vi "Plugin-002-CalibrationTest.vi"(0 "Configuration Page":refnum<class "Material-ConfigPage.lvclass">, 11 "error in":errorcluster) -> (15 "error out":errorcluster)   [LabVIEW 2013, in "Calibration-RunTest.lvclass"]
doc: "DisplayName=\"Deploy Configuration Template\"\nDescription=\"This VI serves as a template page for the Deploy Configuration UI.\""
uses:
  Plugins/Run Calibration Test/Calibration-RunTest.lvclass
  Material-ConfigPage.lvclass
  Reuse Library/featherweight/Core/Sequencer/FTW-Sequencer.lvclass/FTW-Sequencer.ctl
  Plugins/Run Calibration Test/Calibration-RunTest.lvclass/Calibration-RunTest.ctl
  <vilib>/Utility/miscctls.llb/LVPointTypeDef.ctl
  Reuse Library/featherweight/Core/Regex/FTW-Regex.vi
  Reuse Library/featherweight/Core/Error/FTW-ERR-StatusException.vi
  Reuse Library/featherweight/Core/Error/FTW-ERR-ThrowError.vi
  Reuse Library/featherweight/Core/Sequencer/FTW-Sequencer.lvclass
  Reuse Library/featherweight/Core/Messaging/Message.Actor/FTW-Message-Actor.lvclass
  Plugins/Motion Control/Motion-ControlAll.lvclass
  <instrlib>/Keyence LK-G5000/Keyence LK-G5000.lvlib
  <instrlib>/Keyence LK-G5000/Public/Constant/Comm Interface.ctl
  <vilib>/addons/_LabVIEW Style Book/Utilities/Style Book Utilities.lvlib
panel:
  out "Calibration Complete":bool
  in  "Collect Cal Data":bool
  out "Line 3 Calibration Data":dbl[](graph)
  out "Line 2 Calibration Data":dbl[](graph)
  out "Line 1 Calibration Data":dbl[](graph)
  # "Inputs"
  # "Outputs"
  # "Second Plugin"
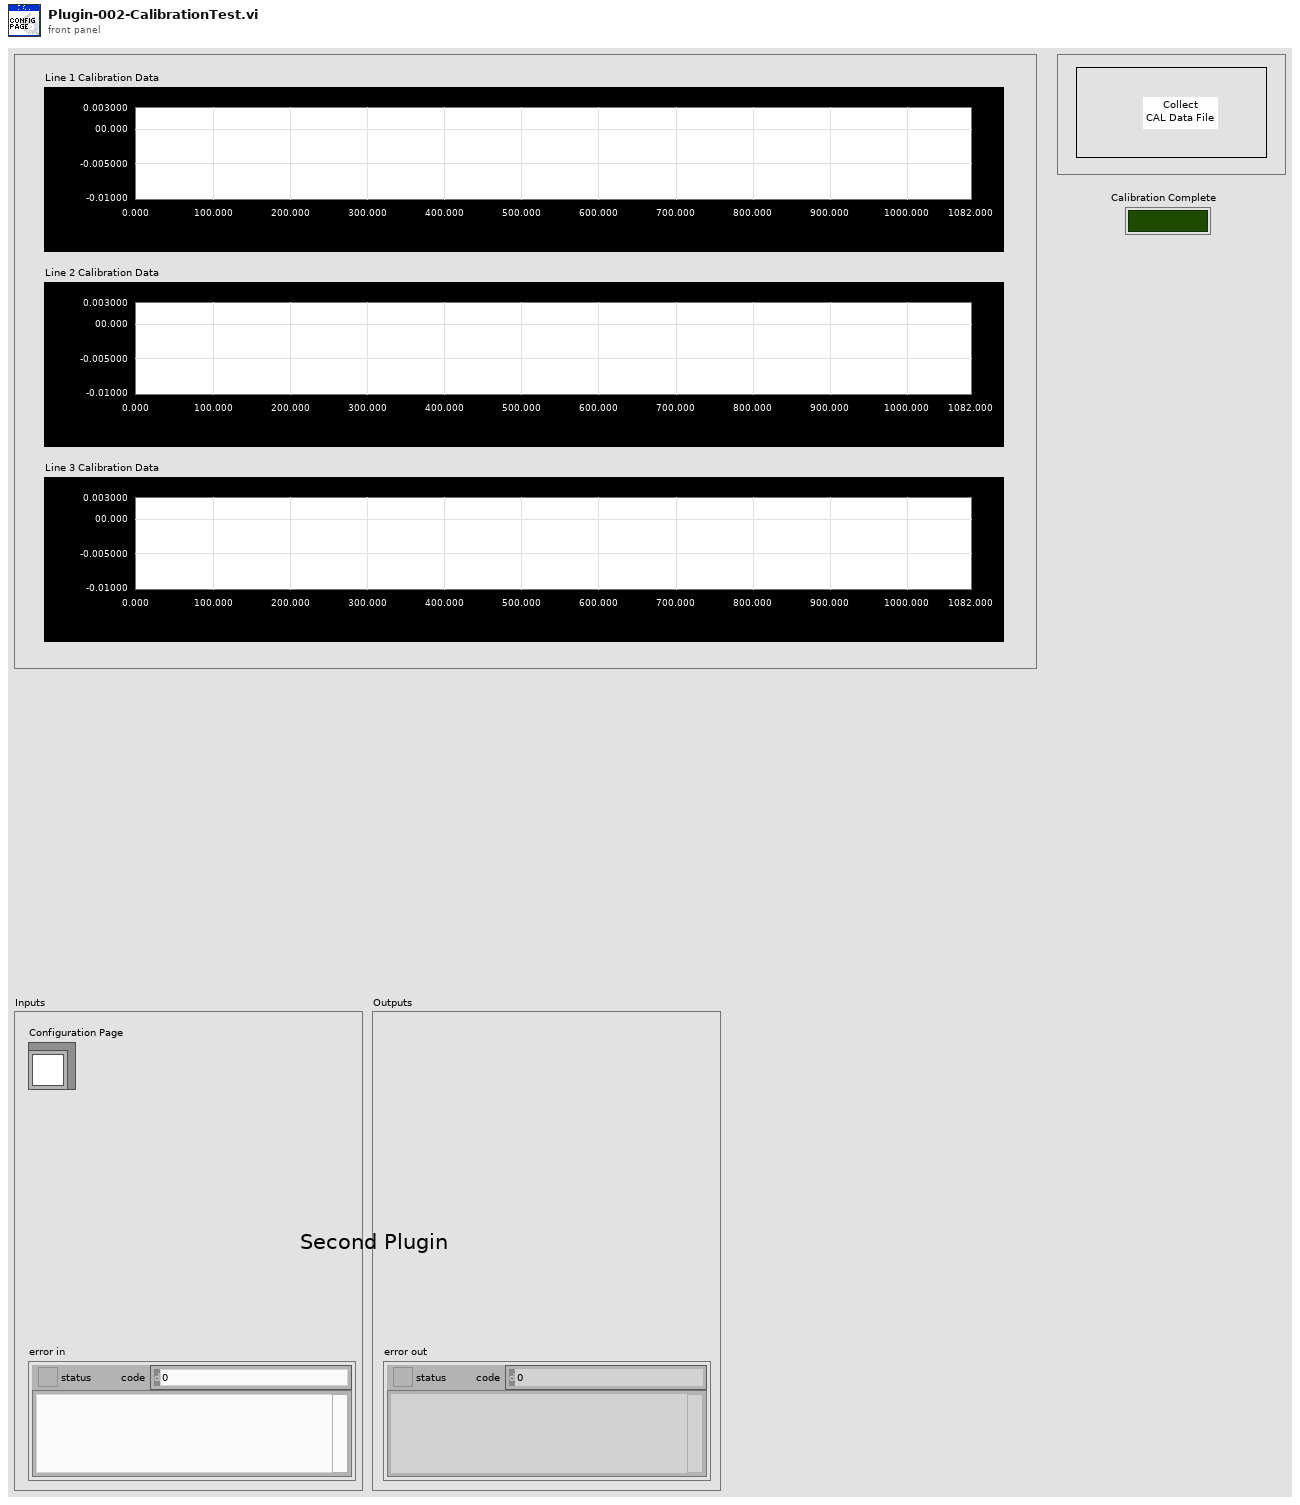
[diagram p1: front panel]
types:
  T1 = typedef "Keyence LK-G5000.lvlib/Comm Interface.ctl" = enum8{"USB", "ETHERNET"}
  T2 = typedef "LVPointTypeDef.ctl" = cluster{"Horizontal":i16, "Vertical":i16}
  T3 = cluster{"PageCommands":refnum<event-registration>}
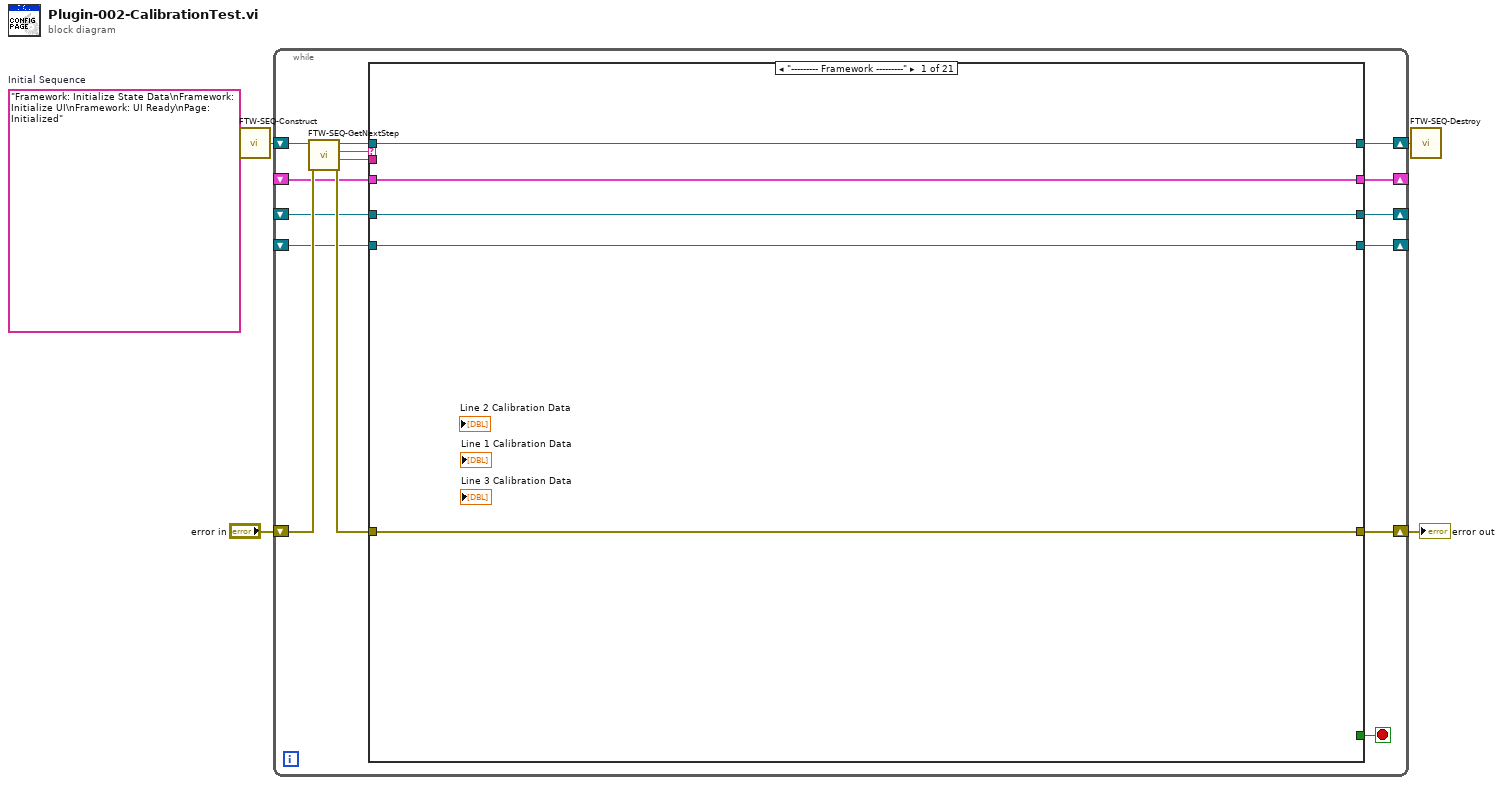
[diagram p0: block diagram]
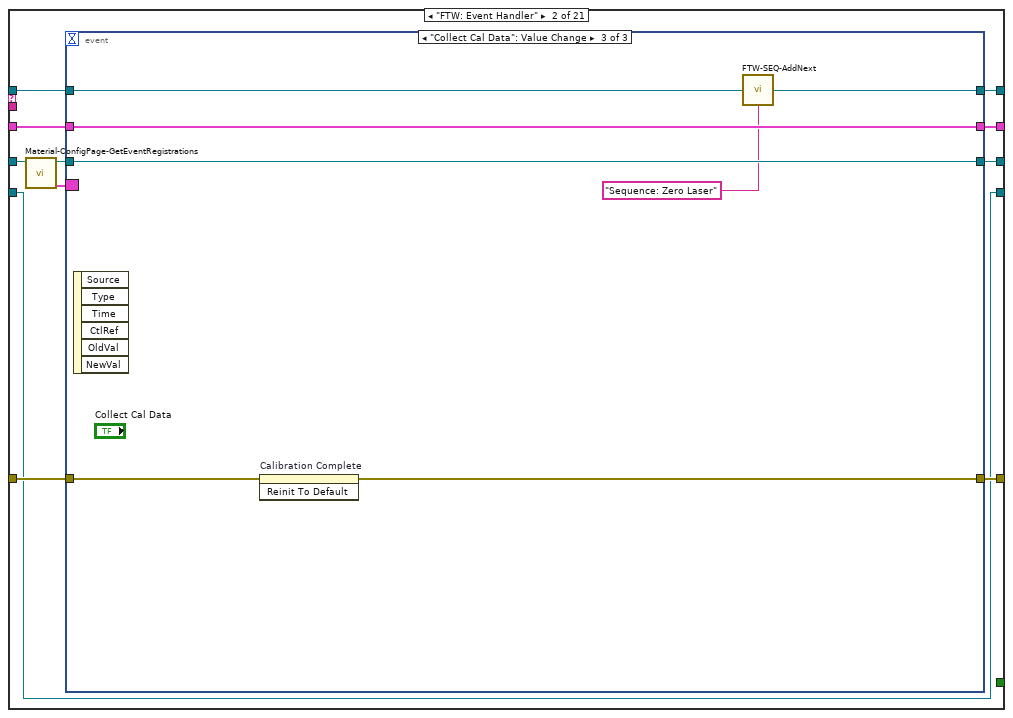
[diagram p2: hidden frame]
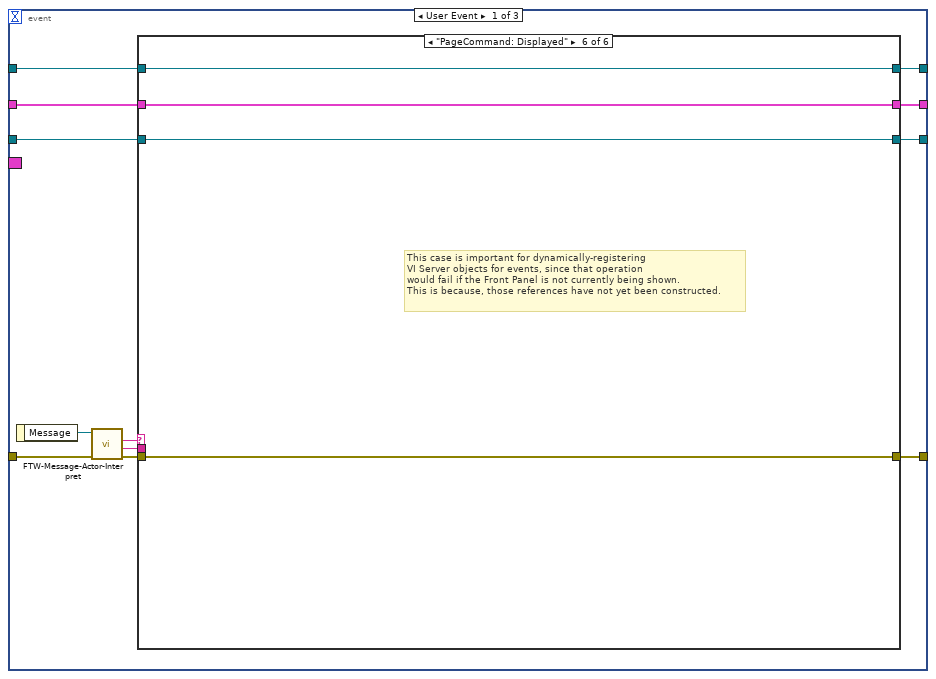
[diagram p3: hidden frame]
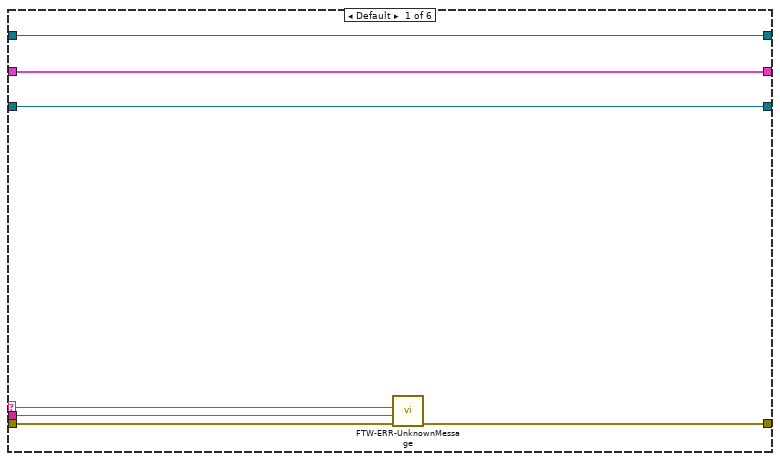
[diagram p4: hidden frame]
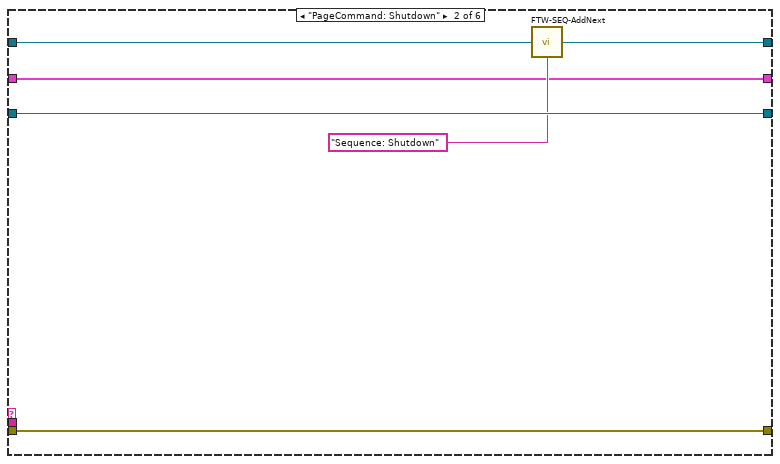
[diagram p5: hidden frame]
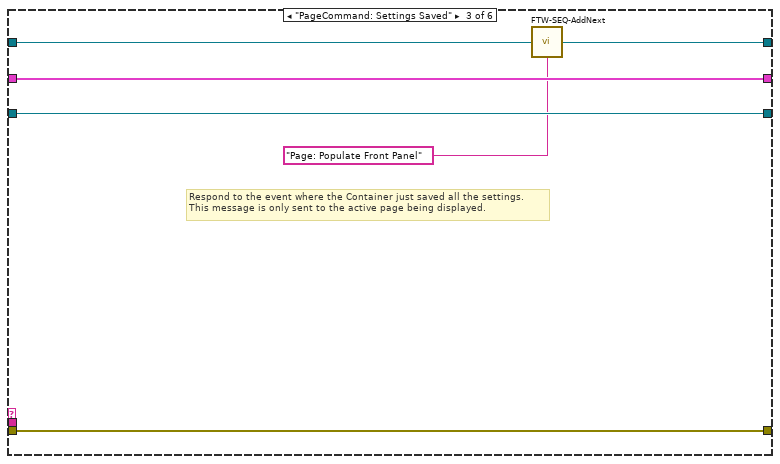
[diagram p6: hidden frame]
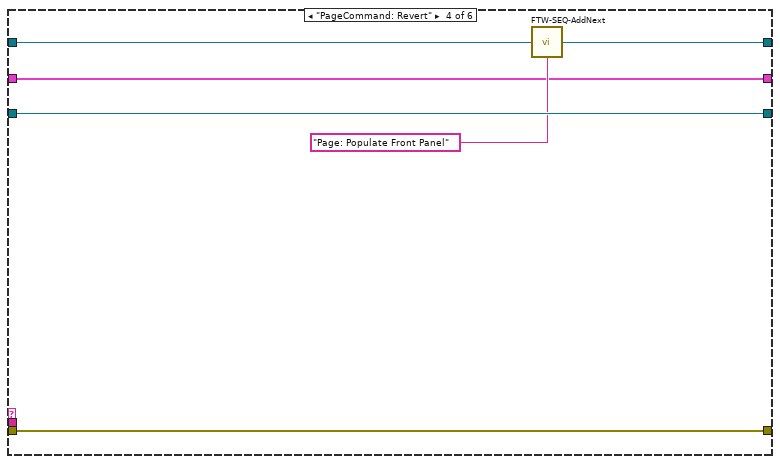
[diagram p7: hidden frame]
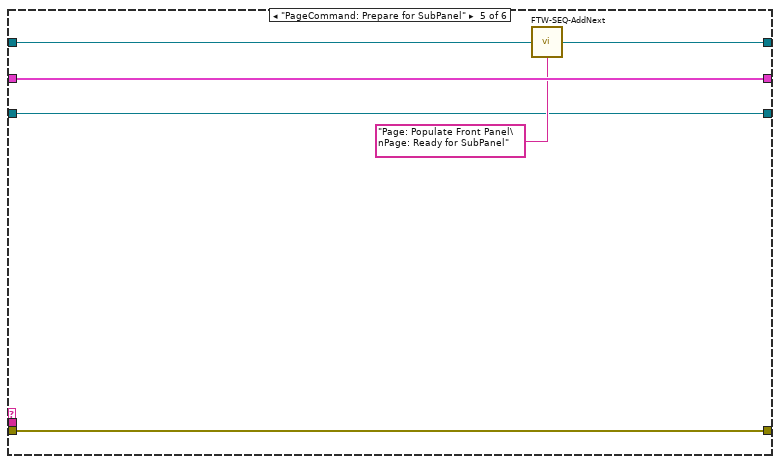
[diagram p8: hidden frame]
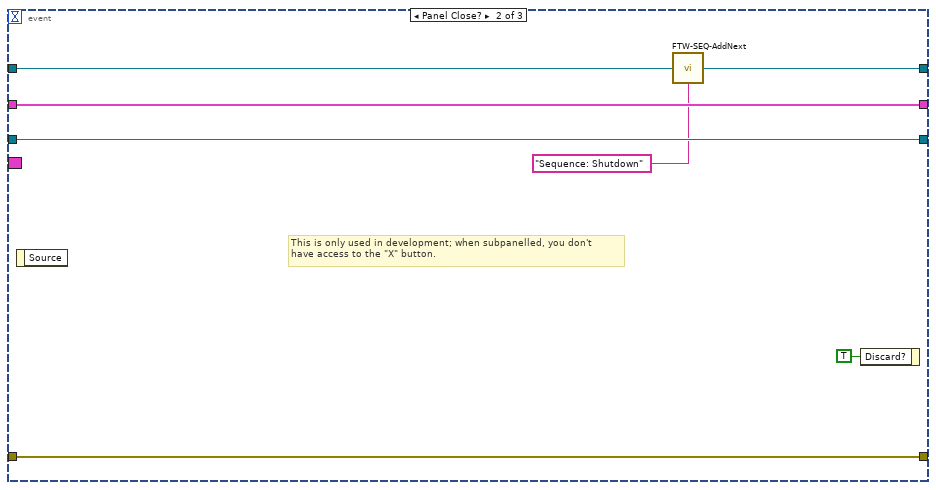
[diagram p9: hidden frame]
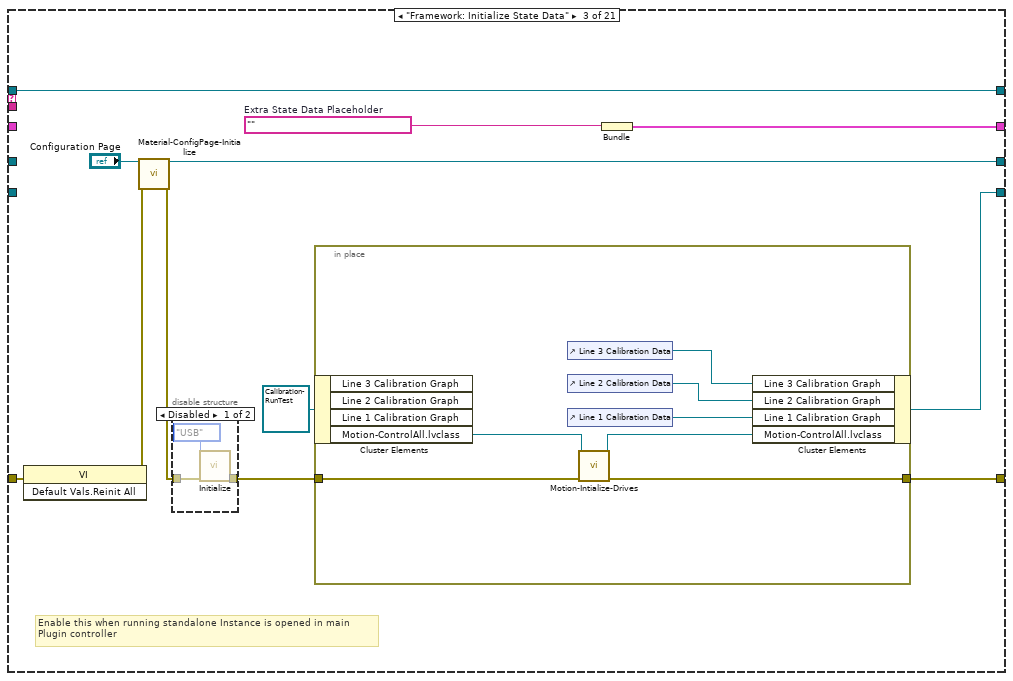
[diagram p10: hidden frame]
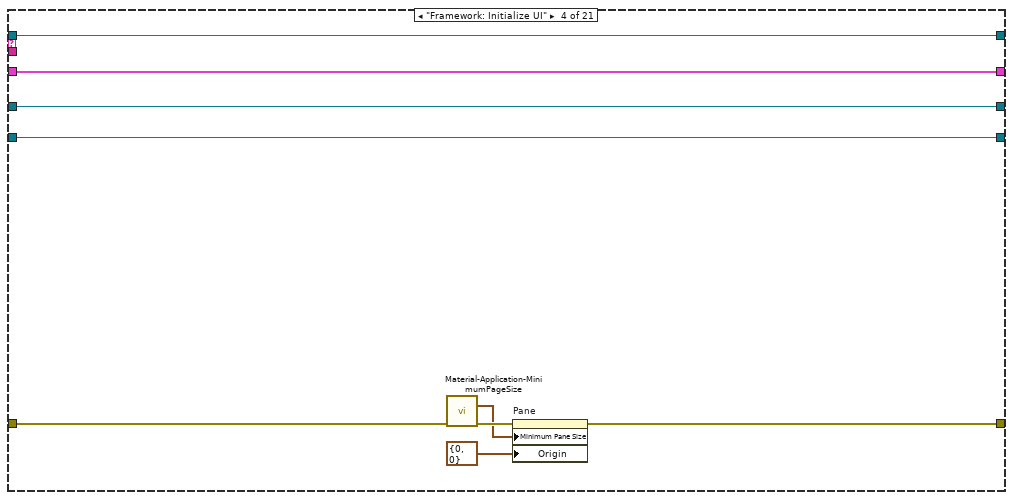
[diagram p12: hidden frame]
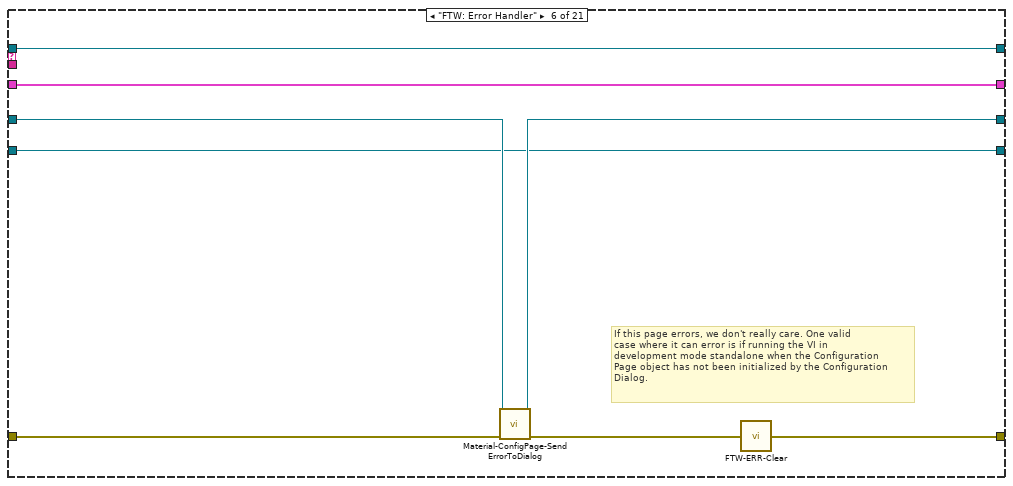
[diagram p14: hidden frame]
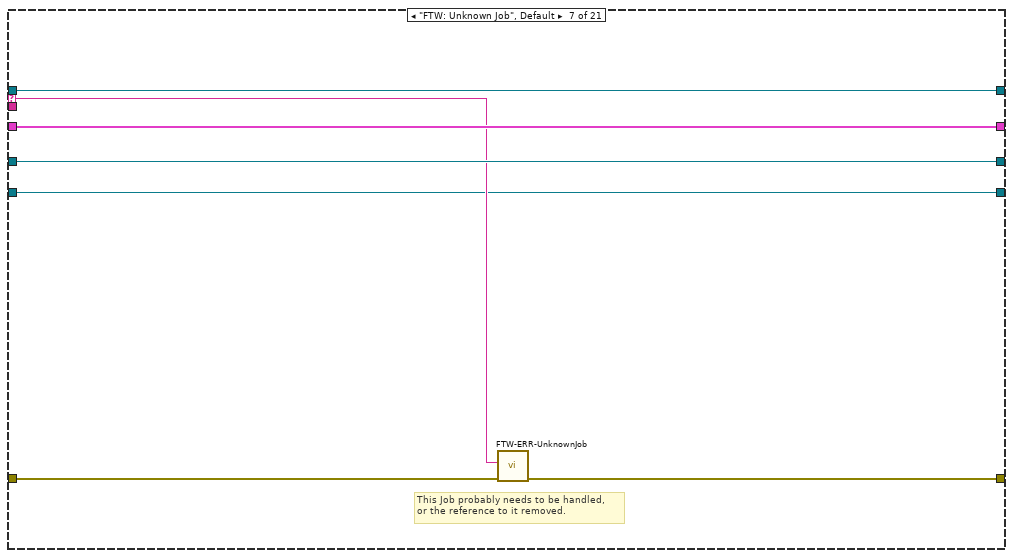
[diagram p15: hidden frame]
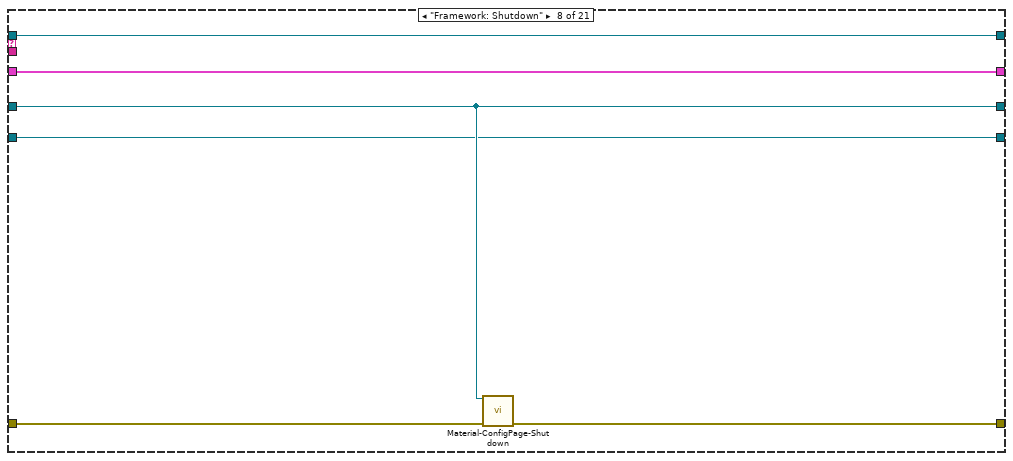
[diagram p16: hidden frame]
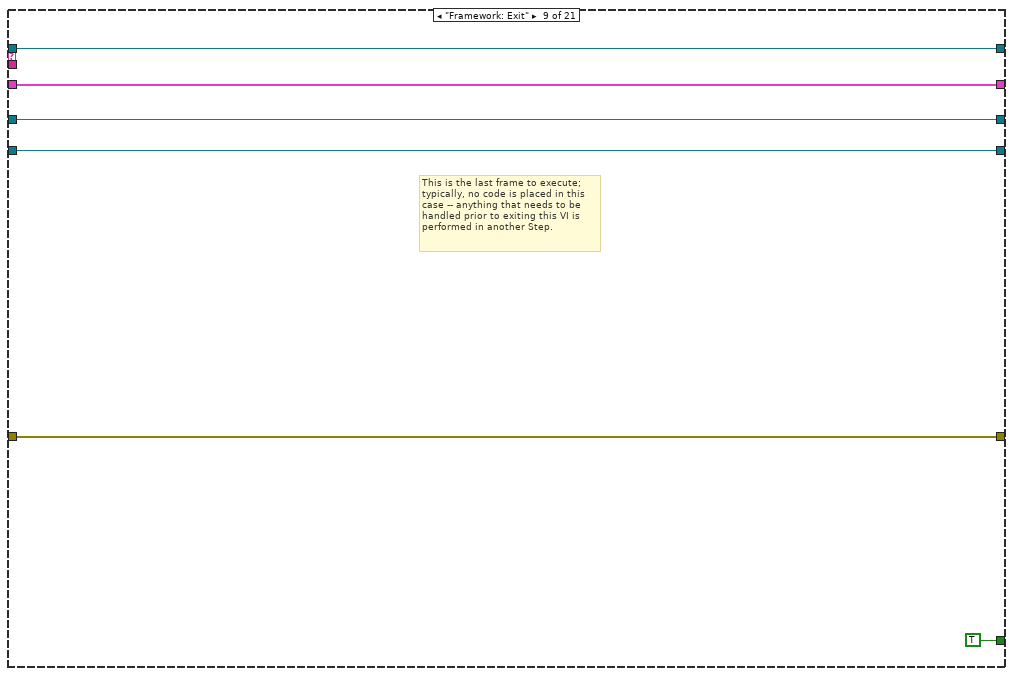
[diagram p17: hidden frame]
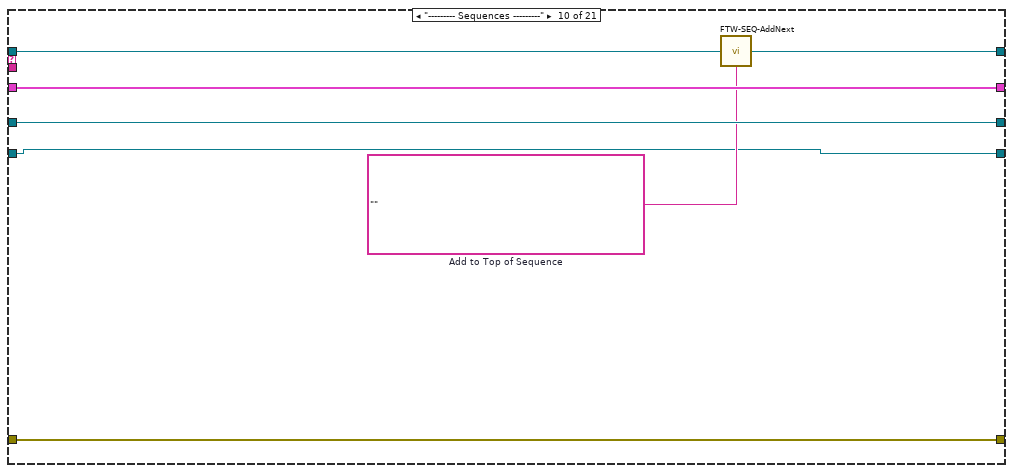
[diagram p18: hidden frame]
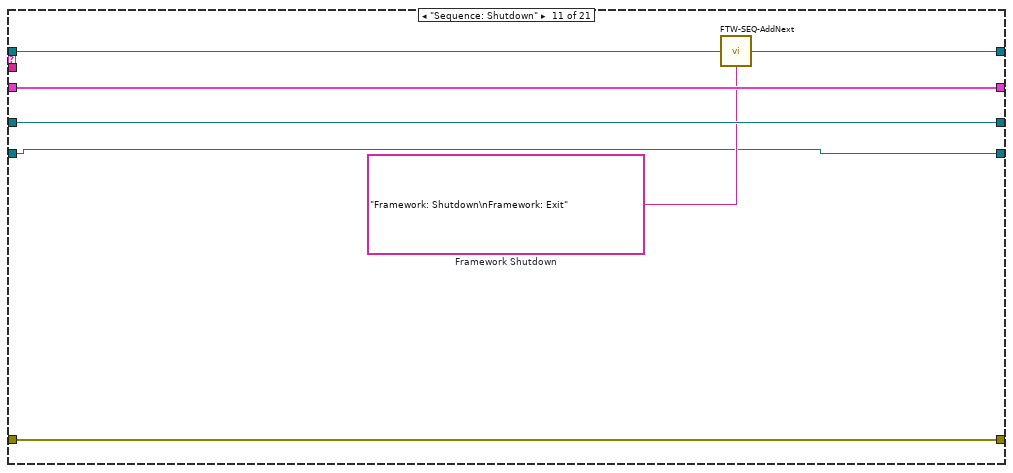
[diagram p19: hidden frame]
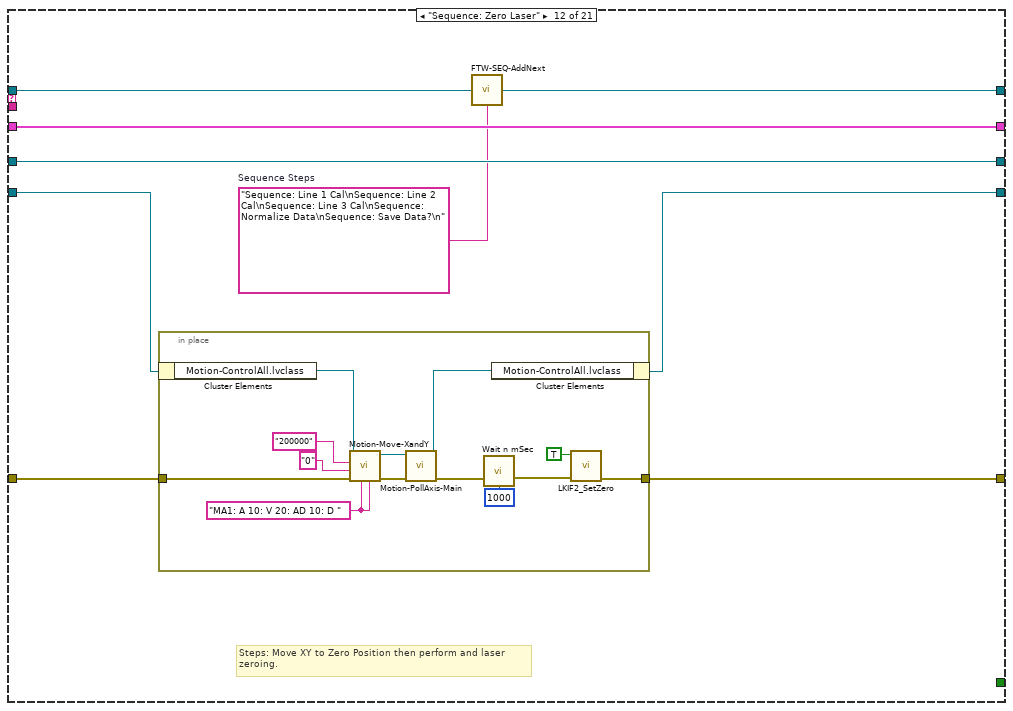
[diagram p20: hidden frame]
diagram:
  w5 = "Framework: Initialize State Data\nFramework: Initialize UI\nFramework: UI Ready\nPage: Initialized"  # Initial Sequence
  n1 = call "FTW-SEQ-Construct.vi"("Initial Sequence"=w5) -> ("Sequencer"=w4:refnum<class "FTW-Sequencer.lvclass">)
  n2 = while {
    shift-right: [w18] -> w3
    shift-left: w4 -> [w9]
    shift-right: [w19] -> w2
    shift-left: "error in" -> [w17]
    shift-right: [w13] -> _
    shift-left: _ -> [w12]
    shift-right: [w11] -> _
    shift-left: _ -> [w10]
    shift-right: [w7] -> _
    shift-left: _ -> [w6]
    stop <- w14 stop-if-true
    n3 = call "FTW-SEQ-GetNextStep.vi"("error in"=w17, "Sequencer"=w9) -> ("error out"=w20:errorcluster, "Job Data"=w8:string, "Current Job"=w15:string, "Sequencer out"=w16:refnum<class "FTW-Sequencer.lvclass">)  [unwired: 6 in]
    n4 = case shown="\"--------- Framework ---------\"" w15 {
      selector: w15 -> [_ _ _ _ _ _ w144 _ _ _ _ _ _ _ _ _ _ _ _ _ _]
      tunnel: [w23 w34 w99 w124 w134 w141 w146 w152 w159 w167 w174 w178 w198 w205 w212 w223 w230 w239 w245 w249 w258] -> w19
      tunnel: w20 -> [w23 w33 w103 w125 w134 w138 w147 w153 w159 w167 w174 w179 w201 w208 w215 w220 w231 w239 w246 w249 w259]
      tunnel: w16 -> [w24 w36 w108 w123 w131 w136 w149 w154 w157 w164 w171 w181 w204 w211 w218 w226 w234 w236 w242 w252 w254]
      tunnel: [w24 w35 w108 w123 w131 w136 w149 w154 w157 w163 w170 w180 w204 w211 w218 w226 w234 w236 w242 w252 w254] -> w18
      tunnel: [_ _ _ _ _ _ _ _ TRUE _ _ _ _ _ _ _ _ _ _ _ _] -> w14
      tunnel: [w25 w32 w109 w129 w133 w142 w148 w155 w160 w168 w175 w184 w203 w210 w217 w225 w233 w238 w247 w251 w257] -> w13
      tunnel: w12 -> [w25 w30 _ w129 w133 w142 w148 w155 w160 w168 w175 w184 w203 w210 w217 w225 w233 w238 w247 w251 w257]
      tunnel: [w22 w31 w107 w128 w132 w139 w145 w151 w158 w166 w173 w183 w202 w209 w216 w224 w232 w237 w243 w250 w255] -> w11
      tunnel: w10 -> [w22 w29 _ w128 w132 w140 w145 w151 w158 w166 w173 w183 w202 w209 w216 w224 w232 w237 w244 w250 w256]
      tunnel: w8 -> [_ _ _ _ _ _ _ _ _ _ _ _ _ _ _ _ _ _ _ _ _]
      tunnel: [w21 w26 w98 w121 w130 w135 w143 w150 w156 w162 w169 w176 w199 w206 w213 w221 w228 w235 w240 w248 w253] -> w7
      tunnel: w6 -> [w21 w26 _ w121 w130 w135 w143 w150 w156 w162 w169 w177 w200 w207 w214 w222 w229 w235 w240 w248 w253]
      frame "--------- Framework ---------" {
      }
      frame "FTW: Event Handler" {
        n5 = call "Material-ConfigPage-GetEventRegistrations.vi"("Configuration Page"=w29) -> ("Events"=w27:T3, "Configuration Page out"=w28:refnum<class "Material-ConfigPage.lvclass">)  [unwired: 9 in]
        n6 = event shown="[2] \"Collect Cal Data\": Value Change" {
          selector: w27 -> [_ _ _]
          dyn-events: _ -> [_ _ _]
          timeout: _ -> [_ _ _]
          tunnel: w36 -> [w42 w85 w93]
          tunnel: [w43 w84 w94] -> w35
          tunnel: [w47 w88 w91] -> w34
          tunnel: w33 -> [w48 w88 w92]
          tunnel: [w41 w89 w96] -> w32
          tunnel: w30 -> [w40 w89 w96]
          tunnel: w28 -> [w45 w87 w97]
          tunnel: [w44 w87 w97] -> w31
          event User Event {
            n7 = event-data() -> ("Message"=w38:refnum<class "FTW-Message.lvclass">)  [unwired: 1 in]
            n8 = call "FTW-Message-Actor-Interpret.vi"("error in"=w48, "Message"=w38) -> ("error out"=w46:errorcluster, "Sender"=w37:string, "Parameter"=w39:string)  [unwired: 6 in, 1 out]
            n9 = case shown="\"PageCommand: Displayed\"" w39 {
              selector: w39 -> [w50 _ _ _ _ _]
              tunnel: [w54 w61 w67 w73 w74 w80] -> w47
              tunnel: w46 -> [w55 w61 w67 w73 w74 w80]
              tunnel: w45 -> [w53 w60 w66 w72 w75 w81]
              tunnel: [w53 w60 w66 w72 w75 w81] -> w44
              tunnel: [w52 w56 w64 w70 w78 w82] -> w43
              tunnel: w42 -> [w52 w59 w65 w71 w79 w82]
              tunnel: [w51 w57 w63 w68 w77 w83] -> w41
              tunnel: w40 -> [w51 w57 w63 w68 w77 w83]
              tunnel: w37 -> [w49 _ _ _ _ _]
              frame Default {
                n10 = call "FTW-ERR-UnknownMessage.vi"("error in"=w55, "Sender"=w49, "Unknown Parameter"=w50) -> ("error out"=w54:errorcluster)  [unwired: 8 in]
              }
              frame "PageCommand: Shutdown" {
                n11 = call "FTW-SEQ-AddNext.vi"("Add Next in Sequence"="Sequence: Shutdown", "Sequencer"=w59) -> ("Sequencer out"=w56:refnum<class "FTW-Sequencer.lvclass">)  [unwired: 2 in]
              }
              frame "PageCommand: Settings Saved" {
                # "Respond to the event where the Container just saved all the settings.\nThis message is only sent to the active page being displayed."
                n12 = call "FTW-SEQ-AddNext.vi"("Add Next in Sequence"="Page: Populate Front Panel" ("Add to Top of Sequence"), "Sequencer"=w65) -> ("Sequencer out"=w64:refnum<class "FTW-Sequencer.lvclass">)  [unwired: 2 in]
              }
              frame "PageCommand: Revert" {
                n13 = call "FTW-SEQ-AddNext.vi"("Add Next in Sequence"="Page: Populate Front Panel", "Sequencer"=w71) -> ("Sequencer out"=w70:refnum<class "FTW-Sequencer.lvclass">)  [unwired: 2 in]
              }
              frame "PageCommand: Prepare for SubPanel" {
                n14 = call "FTW-SEQ-AddNext.vi"("Add Next in Sequence"="Page: Populate Front Panel\nPage: Ready for SubPanel", "Sequencer"=w79) -> ("Sequencer out"=w78:refnum<class "FTW-Sequencer.lvclass">)  [unwired: 2 in]
              }
              frame "PageCommand: Displayed" {
                # "This case is important for dynamically-registering\nVI Server objects for events, since that operation\nwould fail if the Front Panel is not currently being shown.\nThis is because, those references have not yet been constructed."
              }
            }
          }
          event Panel Close? {
            # "This is only used in development; when subpanelled, you don't\nhave access to the \"X\" button."
            n15 = event-data() -> ()  [unwired: 1 in, 1 out]
            n16 = call "FTW-SEQ-AddNext.vi"("Add Next in Sequence"="Sequence: Shutdown" ("Add to Top of Queue"), "Sequencer"=w85) -> ("Sequencer out"=w84:refnum<class "FTW-Sequencer.lvclass">)  [unwired: 2 in]
            n17 = event-data("Discard?"=TRUE) -> ()  [unwired: 1 in, 1 out]
          }
          event "Collect Cal Data": Value Change {
            n18 = event-data() -> ()  [unwired: 1 in, 6 out]
            n19 = invoke on="Calibration Complete" class="Bool (strict)" method="Reinit To Default"(error in=w92) -> (error out=w91:errorcluster)  [unwired: 2 in, 2 out]
            n20 = call "FTW-SEQ-AddNext.vi"("Add Next in Sequence"="Sequence: Zero Laser" ("Add to Top of Queue"), "Sequencer"=w93) -> ("Sequencer out"=w94:refnum<class "FTW-Sequencer.lvclass">)  [unwired: 2 in]
          }
        }
      }
      frame "Framework: Initialize State Data" {
        w106 = ""  # Extra State Data Placeholder
        # "Enable this when running standalone Instance is opened in main\nPlugin controller"
        n21 = invoke class="VI" method="Default Vals.Reinit All"(error in=w103) -> (error out=w102:errorcluster)  [unwired: 2 in, 2 out]
        n22 = call-dynamic "Material-ConfigPage-Initialize.vi"("Configuration Page"="Configuration Page", "error in"=w102) -> ("Configuration Page out"=w107:refnum<class "Material-ConfigPage.lvclass">, "error out"=w104:errorcluster)  [unwired: 12 in]
        n23 = disable-structure shown="Disabled" {
          disable-tunnel: w104 -> [w118 w120]
          disable-tunnel: [w117 w120] -> w100
          frame Disabled {
            n24 = call <instrlib>:"Initialize.vi"("error in (no error)"=w118, "Comm Interface"=Comm_Interface."USB") -> ("error out"=w117:errorcluster)  [unwired: 9 in]
          }
          frame Enabled {
          }
        }
        n25 = in-place {
          in-place-border: w100 -> [w112]
          in-place-border: [w110] -> w99
          n26 = in-place-cluster #1(refnum<class "Calibration-RunTest.lvclass"> refnum ("Calibration-RunTest.lvclass")) -> ("Motion-ControlAll.lvclass"=w113:refnum<class "Motion-ControlAll.lvclass">)  [unwired: 3 out]
          n27 = control-ref of="Line 3 Calibration Data"() -> (w114:refnum<vi>)
          n28 = control-ref of="Line 2 Calibration Data"() -> (w115:refnum<vi>)
          n29 = control-ref of="Line 1 Calibration Data"() -> (w116:refnum<vi>)
          n30 = call "Motion-Intialize-Drives.vi"("error in (no error)"=w112, "Motion-ControlAll in"=w113) -> ("error out"=w110:errorcluster, "Motion-ControlAll out"=w111:refnum<class "Motion-ControlAll.lvclass">)  [unwired: 8 in]
          n31 = in-place-cluster #1("Line 3 Calibration Graph"=w114, "Line 2 Calibration Graph"=w115, "Line 1 Calibration Graph"=w116, "Motion-ControlAll.lvclass"=w111) -> (w98:refnum<class "Calibration-RunTest.lvclass">)
        }
        n32 = Bundle("Extra State Data Placeholder"=w106) -> (w109:cluster{"Extra State Data Placeholder":string})  [unwired: 1 in]
      }
      frame "Framework: Initialize UI" {
        n33 = call "Material-Application-MinimumPageSize.vi"("error in"=w125) -> ("Minimum Pane Size"=w126:cluster{"Horizontal":i16, "Vertical":i16}, "error out"=w127:errorcluster)  [unwired: 13 in]
        n34 = property on="Pane" class="Pane"(error in=w127, "Minimum Pane Size"=w126, "Origin"=T2 {"Horizontal"=0, "Vertical"=0}) -> (error out=w124:errorcluster)  [unwired: 1 in, 1 out]
      }
      frame "Framework: UI Ready" {
      }
      frame "FTW: Error Handler" {
        # "If this page errors, we don't really care. One valid\ncase where it can error is if running the VI in\ndevelopment mode standalone when the Configuration\nPage object has not been initialized by the Configuration\nDialog."
        n35 = call "Material-ConfigPage-SendErrorToDialog.vi"("Configuration Page in"=w140, "error in"=w138) -> ("Configuration Page out"=w139:refnum<class "Material-ConfigPage.lvclass">, "error out"=w137:errorcluster)  [unwired: 12 in]
        n36 = call "FTW-ERR-Clear.vi"("error to snuff"=w137) -> ("no error"=w141:errorcluster)
      }
      frame "FTW: Unknown Job", Default {
        # "This Job probably needs to be handled,\nor the reference to it removed."
        n37 = call "FTW-ERR-UnknownJob.vi"("error in"=w147, "Unknown Job"=w144) -> ("error out"=w146:errorcluster)  [unwired: 9 in]
      }
      frame "Framework: Shutdown" {
        n38 = call "Material-ConfigPage-Shutdown.vi"("Configuration Page"=w151, "error in"=w153) -> ("error out"=w152:errorcluster)  [unwired: 13 in]
      }
      frame "Framework: Exit" {
        # "This is the last frame to execute;\ntypically, no code is placed in this\ncase -- anything that needs to be\nhandled prior to exiting this VI is\nperformed in another Step."
      }
      frame "--------- Sequences ---------" {
        w165 = ""  # Add to Top of Sequence
        n39 = call "FTW-SEQ-AddNext.vi"("Add Next in Sequence"=w165, "Sequencer"=w164) -> ("Sequencer out"=w163:refnum<class "FTW-Sequencer.lvclass">)  [unwired: 2 in]
      }
      frame "Sequence: Shutdown" {
        w172 = "Framework: Shutdown\nFramework: Exit"  # Framework Shutdown
        n40 = call "FTW-SEQ-AddNext.vi"("Add Next in Sequence"=w172, "Sequencer"=w171) -> ("Sequencer out"=w170:refnum<class "FTW-Sequencer.lvclass">)  [unwired: 2 in]
      }
      frame "Sequence: Zero Laser" {
        w182 = "Sequence: Line 1 Cal\nSequence: Line 2 Cal\nSequence: Line 3 Cal\nSequence: Normalize Data\nSequence: Save Data?\n"  # Sequence Steps
        # "Steps: Move XY to Zero Position then perform and laser\nzeroing."
        n41 = in-place {
          in-place-border: w179 -> [w195]
          in-place-border: [w191] -> w178
          w187 = "MA1: A 10: V 20: AD 10: D " ("concatenated string")
          n42 = in-place-cluster #2(w177) -> ("Motion-ControlAll.lvclass"=w186:refnum<class "Motion-ControlAll.lvclass">)
          n43 = call "Motion-Move-XandY.vi"("Y Drive Acc/Speed/Velocity"=w187, "X Drive Acc/Speed/Velocity"=w187, "error in (no error)"=w195, "X Coordinates"="0", "Y Coordinates"="200000", "Motion-ControlAll in"=w186) -> ("error out"=w193:errorcluster, "Motion-ControlAll out"=w194:refnum<class "Motion-ControlAll.lvclass">)  [unwired: 4 in]
          n44 = call "Motion-PollAxis-Main.vi"("error in (no error)"=w193, "Motion-ControlAll in"=w194) -> ("error out"=w190:errorcluster, "Motion-ControlAll out"=w185:refnum<class "Motion-ControlAll.lvclass">)  [unwired: 8 in]
          n45 = call <vilib>:"Wait n mSec.vi"("error in (no error)"=w190, "Milliseconds to Wait (500)"=u32 1000) -> ("error out"=w188:errorcluster)  [unwired: 13 in]
          n46 = in-place-cluster #2("Motion-ControlAll.lvclass"=w185) -> (w176:refnum<class "Calibration-RunTest.lvclass">)
          n47 = call <instrlib>:"LKIF2_SetZero.vi"("error in (no error)"=w188, "OnOff"=TRUE) -> ("error out"=w191:errorcluster)  [unwired: 9 in]
        }
        n48 = call "FTW-SEQ-AddNext.vi"("Add Next in Sequence"=w182, "Sequencer"=w181) -> ("Sequencer out"=w180:refnum<class "FTW-Sequencer.lvclass">)  [unwired: 2 in]
      }
      frame "Sequence: Line 1 Cal" {
        n49 = call "Calibration-Line1-CalMain.vi"("error in (no error)"=w201, "Calibration-RunTest in"=w200) -> ("error out"=w198:errorcluster, "Calibration-RunTest out"=w199:refnum<class "Calibration-RunTest.lvclass">)  [unwired: 8 in]
      }
      frame "Sequence: Line 2 Cal" {
        n50 = call "Calibration-Line2-CalMain.vi"("error in (no error)"=w208, "Calibration-RunTest in"=w207) -> ("error out"=w205:errorcluster, "Calibration-RunTest out"=w206:refnum<class "Calibration-RunTest.lvclass">)  [unwired: 8 in]
      }
      frame "Sequence: Line 3 Cal" {
        n51 = call "Calibration-Line3-CalMain.vi"("error in (no error)"=w215, "Calibration-RunTest in"=w214) -> ("error out"=w212:errorcluster, "Calibration-RunTest out"=w213:refnum<class "Calibration-RunTest.lvclass">)  [unwired: 8 in]
      }
      frame "Sequence: Normalize Data" {
        n52 = call "Calibration-Splash-Normalizing.vi"("error in (no error)"=w220) -> ("error out"=w219:errorcluster)  [unwired: 10 in]
        n53 = call "Calibration-NormalizeData.vi"("error in (no error)"=w219, "Calibration-RunTest in"=w222) -> ("error out"=w223:errorcluster, "Calibration-RunTest out"=w221:refnum<class "Calibration-RunTest.lvclass">)  [unwired: 8 in]
      }
      frame "Sequence: Save Data?" {
        n54 = call "Calibration-SaveData.vi"("error in (no error)"=w231, "Calibration-RunTest in"=w229) -> ("error out"=w230:errorcluster, "Cal Finished"=→"Calibration Complete":bool, "Calibration-RunTest out"=w228:refnum<class "Calibration-RunTest.lvclass">)  [unwired: 7 in]
      }
      frame "--------- Application Logic ---------" {
      }
      frame "Page: Initialized" {
        w241 = TRUE  # Allow user to open Diagram from SubPanel?
        n55 = call "Material-ConfigPage-Initialized.vi"("Configuration Page"=w244, "Allow user to open Diagram from SubPanel?"=w241, "error in"=w246) -> ("Configuration Page out"=w243:refnum<class "Material-ConfigPage.lvclass">, "error out"=w245:errorcluster)  [unwired: 11 in]
      }
      frame "Page: Populate Front Panel" {
      }
      frame "Page: Ready for SubPanel" {
        n56 = call "Material-ConfigPage-ReadyForSubPanel.vi"("Configuration Page"=w256, "error in"=w259) -> ("Configuration Page out"=w255:refnum<class "Material-ConfigPage.lvclass">, "error out"=w258:errorcluster)  [unwired: 12 in]
      }
    }
  }
  "error out" <- w2
  n57 = call "FTW-SEQ-Destroy.vi"("Sequencer"=w3) -> ()  [unwired: 1 in]
